vi "LabVIEW version alias to path.vi"(8 "error in (no error)":errorcluster, 11 "LabVIEW version string":string) -> (0 "error out":errorcluster, 3 "LabVIEW path":path)   [LabVIEW 2021]
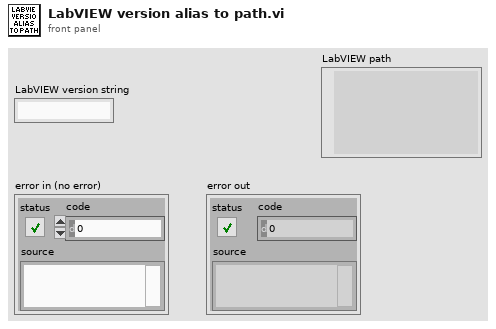
[diagram p1: front panel]
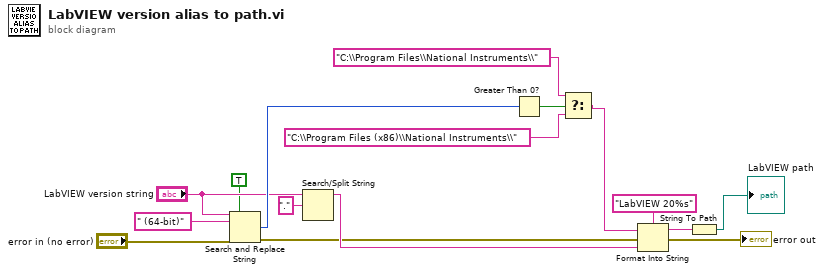
[diagram p0: block diagram]
diagram:
  n1 = Search and Replace String(replace all?=TRUE ("replace all? (F)"), input string="LabVIEW version string", search string=" (64-bit)", error in="error in (no error)") -> (number of replacements=w15:i32, error out=w8:errorcluster)  [unwired: 4 in, 2 out]
  n2 = Search/Split String(string="LabVIEW version string", search string/char (-)=".") -> (substring before match=w10:string)  [unwired: 1 in, 2 out]
  n3 = Greater Than 0?(x=w15) -> (x > 0?=w14:bool)
  n4 = Select(t="C:\\Program Files\\National Instruments\\" ("input string"), s=w14, f="C:\\Program Files (x86)\\National Instruments\\" ("input string")) -> (s? t:f=w6:string)
  n5 = Format Into String(format string="LabVIEW 20%s", initial string=w6, error in=w8, w10) -> (resulting string=w2:string, error out=→"error out":errorcluster)
  n6 = String To Path(string=w2) -> (path=→"LabVIEW path":path)
